vi "enable joystick.vi"() -> (3 "元素":dbl)   [LabVIEW 2014]
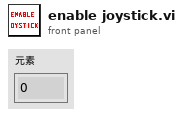
[diagram p1: front panel]
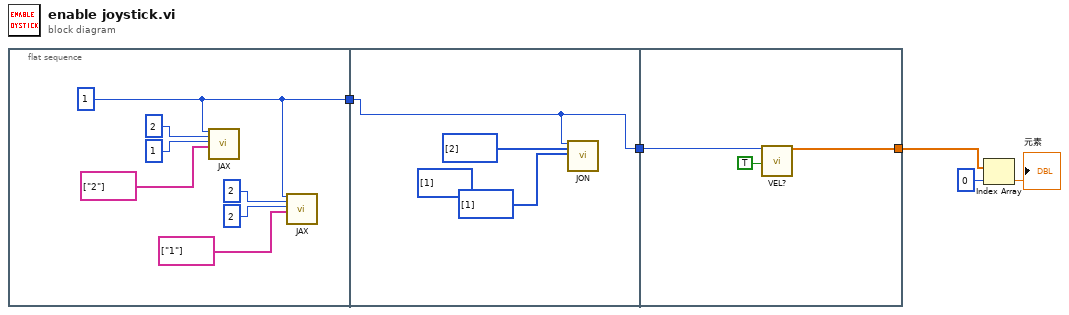
[diagram p0: block diagram]
diagram:
  (unwired) i32[] [1] ("Joystick mode")
  n1 = flat-sequence {
    tunnel: [w6] -> w5
    tunnel: w5 -> [w13]
    tunnel: [w13] -> w4
    tunnel: w4 -> [w18]
    tunnel: [w17] -> w2
    frame #0 {
      w6 = 1 ("System no.")
      n2 = call "JAX.vi"("System no."=w6, "JoystickID"=2 ("Joystick axis"), "Joystick axis"=1 ("JoystickID"), "Axes to set"=string[] ["2"]) -> ()  [unwired: 15 in, 1 out]
      n3 = call "JAX.vi"("System no."=w6, "JoystickID"=2 ("Joystick axis"), "Joystick axis"=2 ("JoystickID"), "Axes to set"=string[] ["1"]) -> ()  [unwired: 15 in, 1 out]
    }
    frame #1 {
      n4 = call "JON.vi"("System no."=w13, "JoystickID to set"=i32[] [2], "Joystick mode"=i32[] [1]) -> ()  [unwired: 15 in, 2 out]
    }
    frame #2 {
      n5 = call "VEL?.vi"("System no."=w18, "All axes?"=TRUE) -> ("Velocity"=w17:dbl[])  [unwired: 16 in, 1 out]
    }
  }
  n6 = Index Array(array=w2, index=0 ("索引")) -> (element=→"元素":dbl)
